vi "subExpandAndFindExternalDeps.vi"(11 "PATH in":string) -> (3 "Expanded deps":path[](array[path]))   [LabVIEW 2019, in "SolutionBuilder.lvlib" / "SolutionBuilder.lvclass"]
uses:
  SolutionBuilder.lvclass
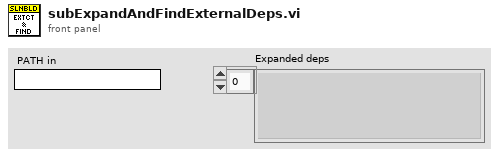
[diagram p1: front panel]
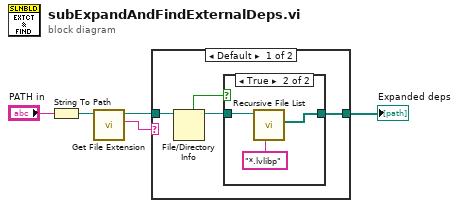
[diagram p0: block diagram]
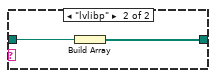
[diagram p3: hidden frame]
diagram:
  n1 = String To Path(string="PATH in") -> (path=w4:path)
  n2 = call <vilib>:"Get File Extension.vi"("file"=w4) -> ("lowercase file extension"=w2:string, "dup file"=w3:path)  [unwired: 6 in, 3 out]
  n3 = case shown="Default" w2 {
    tunnel: w3 -> [w6 w14]
    tunnel: [w7 w13] -> w1
    frame Default {
      n4 = File/Directory Info(path=w6) -> (path out=w8:path, directory=w9:bool)  [unwired: 1 in, 5 out]
      n5 = case shown="True" w9 {
        tunnel: w8 -> [_ w12]
        tunnel: [_ w10] -> w7
        frame False {
        }
        frame True {
          n6 = call <vilib>:"Recursive File List.vi"("pattern"="*.lvlibp", "Folder Path"=w12) -> ("All Files in Dir"=w10:path[])  [unwired: 5 in, 4 out]
        }
      }
    }
    frame "lvlibp" {
      n7 = Build Array(w14) -> (w13:path[])
    }
  }
  "Expanded deps" <- w1
